vi "Send Data.vi"(8 "error in (no error)":errorcluster, 11 "Rigol DG822 Square in":refnum<class "Rigol DG822 Square.lvclass">) -> (0 "error out":errorcluster, 3 "Rigol DG822 Square out":refnum<class "Rigol DG822 Square.lvclass">)   [LabVIEW 2021, in "Rigol DG822 UI.lvlib" / "Rigol DG822 Square.lvlib" / "Rigol DG822 Square.lvclass"]
uses:
  Rigol DG822 Square.lvclass
  Rigol DG822 UI/lib/controls.llb/RDG822ExtCall.ctl
  Rigol DG822 Square.lvclass/Rigol DG822 Square.ctl
  <userlib>/_MGI/Timing/MGI Wait/MGI Wait (U32).vi
  General/Files/lvlibp/Actors.lvlibp/Actors/Actors/Actors.lvclass
  D:/LabVIEW/General/Files/lvlibp/Actors.lvlibp/Actors/Actors/Actors.lvclass
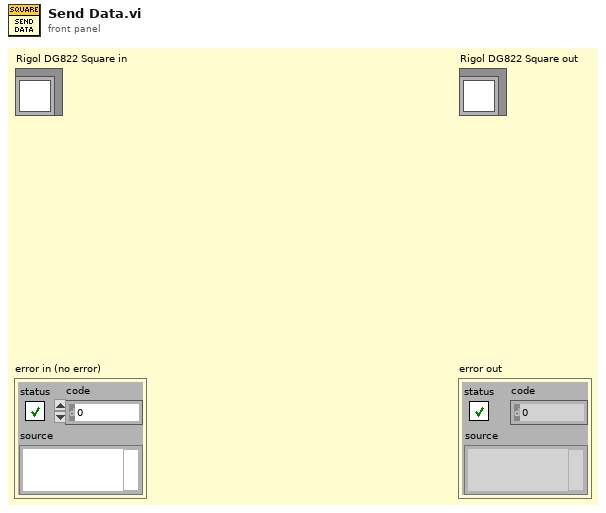
[diagram p1: front panel]
types:
  T1 = typedef "RDG822ExtCall.ctl" = enum16{"Get Data"}
  T2 = typedef "AllWaveformDataCluster.ctl" = cluster{"Data":T3, "F/T Ctrls":T4, "String Indcs":T5}
  T3 = typedef "DataCluster.ctl" = cluster{"Freq":cluster{"Freq":dbl, "FreqUnit":enum32{"No Selection", "MHz", "kHz", "Hz", "mHz", "uHz"}, "FreqUnitPrcs":dbl}, "Period":cluster{"Period":dbl, "PeriodUnit":enum32{"No Selection", "s", "ms", "us", "ns"}, "PeriodUnitPrcs":dbl}, "Ampl":cluster{"Ampl":dbl, "AmplUnit":enum32{"No Selection", "Vpp", "mVpp"}, "AmplUnitPrcs":dbl}, "HighL":cluster{"HighL":dbl, "HighLUnit":enum32{"No Selection", "V", "mV"}, "HighLUnitPrcs":dbl}, "Offset":cluster{"Offset":dbl, "OffsetUnit":enum32{"No Selection", "Vdc", "mVdc"}, "OffsetUnitPrcs":dbl}, "LowL":cluster{"LowL":dbl, "LowLUnit":enum32{"No Selection", "V", "mV"}, "LowLUnitPrcs":dbl}, "Phase":cluster{"Phase":dbl, "PhaseUnit":enum32{"°"}, "PhaseUnitPrcs":dbl}, "Duty":cluster{"Duty":dbl, "DutyUnit":enum32{"%"}, "DutyUnitPrcs":dbl}, "Width":cluster{"Width":dbl, "WidthUnit":enum32{"No Selection", "s", "ms", "us", "ns"}, "WidthUnitPrcs":dbl}, "RisEdge":cluster{"RisEdge":dbl, "RisEdgeUnit":enum32{"No Selection", "s", "ms", "us", "ns"}, "RisEdgeUnitPrcs":dbl}, "FallEdge":cluster{"FallEdge":dbl, "FallEdgeUnit":enum32{"No Selection", "s", "ms", "us", "ns"}, "FallEdgeUnitPrcs":dbl}}
  T4 = typedef "FT Controls Cluster.ctl" = cluster{"Freq/Period":bool, "Ampl/HighL":bool, "Offset/LowL":bool, "Duty/Width":bool}
  T5 = typedef "String Indicators Cluster.ctl" = cluster{"Freq-Period":string, "Ampl-HighL":string, "Offset-LowL":string, "Phase":string, "Duty-Width":string, "RisEdge":string, "FallEdge":string}
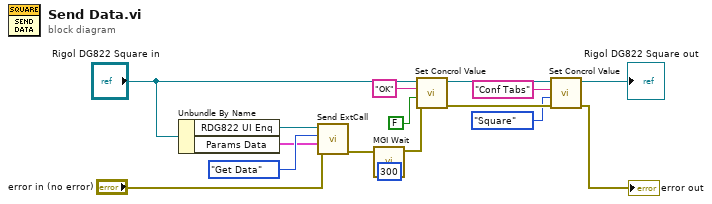
[diagram p0: block diagram]
diagram:
  n1 = Unbundle By Name("Rigol DG822 Square in") -> ("RDG822 UI Enq"=w14:refnum<class "Message Enqueuer.lvclass">, "Params Data"=w13:T2)
  n2 = call "Send ExtCall.vi"("error in (no error)"="error in (no error)", "Val"=w13, "Tag"=RDG822ExtCall."Get Data", "Message Enqueuer"=w14) -> ("error out"=w12:errorcluster)  [unwired: 4 in, 3 out]
  n3 = call-poly <userlib>:"MGI Wait.vi"("ms"=u32 300, "Error In"=w12) -> ("Error Out"=w10:errorcluster)  [unwired: 5 in]
  n4 = call "Set Concrol Value.vi"("error in (no error)"=w10, "Value"=FALSE ("Menu"), "Control Label"="OK", "Actors in"="Rigol DG822 Square in") -> ("error out"=w8:errorcluster, "Actors out"=w7:refnum<class "Rigol DG822 Square.lvclass">)  [unwired: 6 in]
  n5 = call "Set Concrol Value.vi"("error in (no error)"=w8, "Value"=enum32{"Square", "OK"}."Square" ("Conf Tabs"), "Control Label"="Conf Tabs", "Actors in"=w7) -> ("error out"=→"error out":errorcluster, "Actors out"=→"Rigol DG822 Square out":refnum<class "Rigol DG822 Square.lvclass">)  [unwired: 6 in]
